vi "Get Number New Images.vi"(8 "error in (no error)":errorcluster, 11 "CCDCamera in":refnum<class "Simulated_CCD_Camera.lvclass">) -> (0 "error out":errorcluster, 2 "New Images ?":bool, 3 "CCDCamera out":refnum<class "Simulated_CCD_Camera.lvclass">)   [LabVIEW 2018, in "Simulated_CCD_Camera.lvclass"]
uses:
  Simulated_CCD_Camera.lvclass
  Simulated_CCD_Camera.lvclass/Simulated_CCD_Camera.ctl
  Interface/Interface.lvclass/Interface.ctl
  Interface/Interface.lvclass
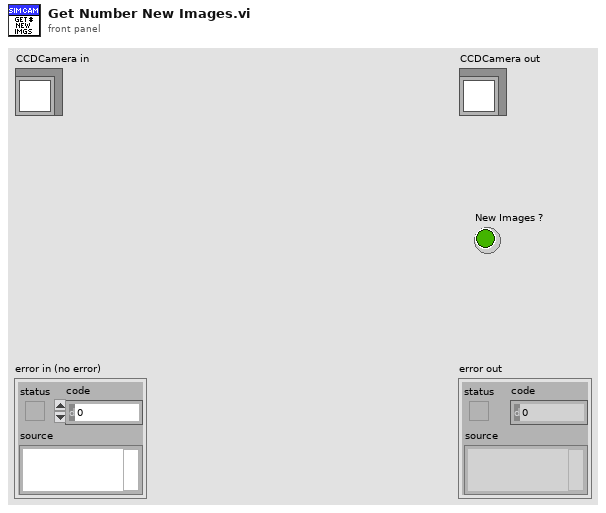
[diagram p1: front panel]
types:
  T1 = cluster{"COOLER_POWER_STATUS":u16, "TEMP":i32, "EXPTIME":dbl, "#FRAMES":u32, "#CUBES":u32}
  T2 = cluster{"CUBE_EXPOSURE_TIME":sgl, "CUBES_DONE":u16, "LAST_IMAGE_NAME":string, "DISK_SPACE":u16, "FRAMES_DONE":u16, "CCD_STATUS":string, "CURRENT_TEMPERATURE":i16, "TEMPERATURE_STATUS":string, "FRAME_EXPOSURE_TIME":dbl, "CCD_POWER_STATUS":bool, "SERIAL_NUMBER":u16, "ACQUIRING":bool}
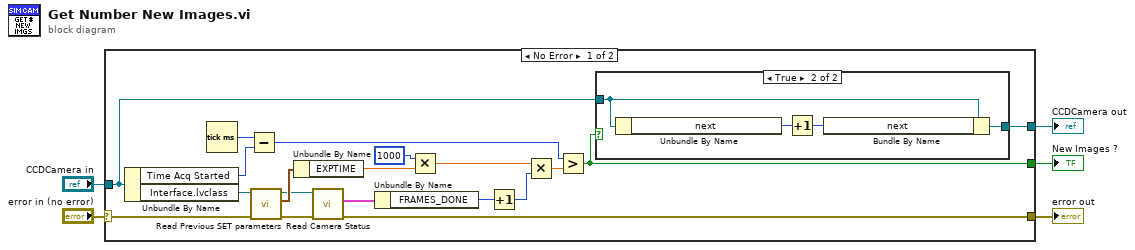
[diagram p0: block diagram]
diagram:
  n1 = case shown="No Error" "error in (no error)" {
    selector: "error in (no error)" -> [w21 w31]
    tunnel: [w7 w31] -> w4
    tunnel: [w24 w30] -> w2
    tunnel: "CCDCamera in" -> [w23 w30]
    tunnel: [w6 _] -> w1
    frame No Error {
      n2 = Unbundle By Name(w23) -> ("Time Acq Started"=w16:u32, "Interface.lvclass"=w22:refnum<class "Interface.lvclass">)
      n3 = Tick Count (ms)() -> (millisecond timer value=w17:u32)
      n4 = Subtract(x=w17, y=w16) -> (x-y=w9:u32)
      n5 = call "Read Previous SET parameters.vi"("error in (no error)"=w21, "Interface in"=w22) -> ("error out"=w15:errorcluster, "Previous SET parameters"=w20:T1, "Interface out"=w14:refnum<class "Interface.lvclass">)  [unwired: 7 in]
      n6 = Unbundle By Name(w20) -> ("EXPTIME"=w19:dbl)
      n7 = call "Read Camera Status.vi"("error in (no error)"=w15, "Interface in"=w14) -> ("error out"=w7:errorcluster, "Camera Status"=w13:T2)  [unwired: 7 in, 1 out]
      n8 = Unbundle By Name(w13) -> ("FRAMES_DONE"=w10:u16)
      n9 = Multiply(x=1000, y=w19) -> (x*y=w12:dbl)
      n10 = Increment(x=w10) -> (x+1=w11:u16)
      n11 = Multiply(x=w12, y=w11) -> (x*y=w8:dbl)
      n12 = Greater?(x=w9, y=w8) -> (0:w6:bool)
      n13 = case shown="True" w6 {
        tunnel: [w25 w29] -> w24
        tunnel: w23 -> [w25 w28]
        frame False {
        }
        frame True {
          n14 = Unbundle By Name(w28) -> ("next"=w27:u16)
          n15 = Increment(x=w27) -> (x+1=w26:u16)
          n16 = Bundle By Name(cluster=w28, "next"=w26) -> (w29:refnum<class "Simulated_CCD_Camera.lvclass">)
        }
      }
    }
    frame Error {
    }
  }
  "error out" <- w4
  "CCDCamera out" <- w2
  "New Images ?" <- w1
